vi "Send Capture Command.vi"(8 "error in (no error)":errorcluster, 10 "nCmd":T1 items=["ACQ_INIT"=0, "DARK_MODE"=1, "BRIGHT_MODE"=2, "SOFTTRIGGER_MODE"=258, "SOFTTRIGGER_INSTANT_MODE"=259], 11 "nSensorIP":u32) -> (0 "error out":errorcluster, 3 "function return":i32)   [LabVIEW 2022 SP3, in "BonTechDetector.lvlib"]
doc: "extern \"C\" BONTECHLIBRARY_API int __stdcall SendCaptureCommand(unsigned int nSensorIP, int nCmd);"
uses:
  BonTechDetector.lvlib
  Controls/Acquisition Commands.ctl
  BonTechWrapperLibrary.dll
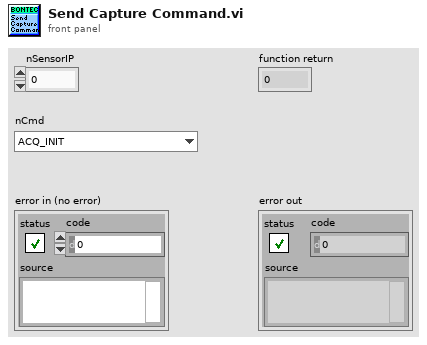
[diagram p1: front panel]
types:
  T1 = typedef "BonTechDetector.lvlib/Acquisition Commands.ctl" = u32
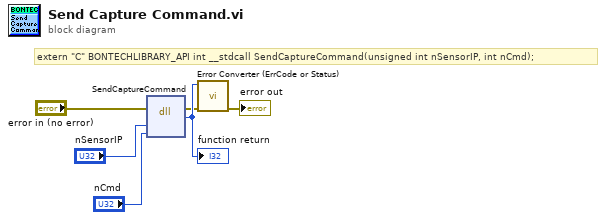
[diagram p0: block diagram]
diagram:
  # "extern \"C\" BONTECHLIBRARY_API int __stdcall SendCaptureCommand(unsigned int nSensorIP, int nCmd);"
  n1 = dll-call lib="E:/Workspace/The-Oracle-feature-highlight-smooth-filter-on-freeze-mode/Image Acquisition/Child Classes/BonTechFlatPanel/BonTechWrapperLibrary.*" fn="SendCaptureCommand"(error in="error in (no error)", "nSensorIP"="nSensorIP", "nCmd"="nCmd") -> (error out=w2:errorcluster, "return type"=w6:i32)  [unwired: 4 in, 1 out]
  "function return" <- w6
  n2 = call "Error Converter (ErrCode or Status).vi"("error in (no error)"=w2, "error code"=w6) -> ("error out"=→"error out":errorcluster)  [unwired: 9 in]
